vi "RampPointsToArray.vi"(6 "Points":dbl, 9 "Distance":dbl, 10 "Range Z":dbl, 11 "Offset":dbl) -> (2 "RampDistancePoints":dbl[][](array[numeric]), 3 "PointsArray":dbl[](array[numeric]))   [LabVIEW 2016]
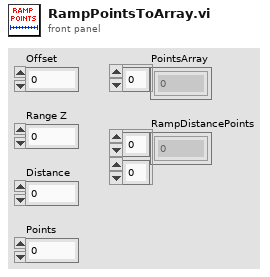
[diagram p1: front panel]
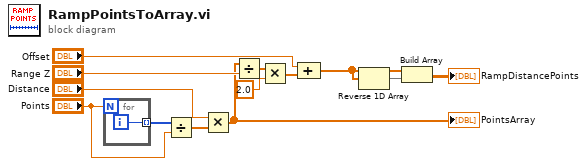
[diagram p0: block diagram]
diagram:
  n1 = for {
    N: "Points" -> [_]
    tunnel: [w14] -> w12 mode=indexing
    i -> [w14]
  }
  n2 = Divide(x=w12, y="Points") -> (x/y=w2:dbl[])
  n3 = Multiply(x="Distance", y=w2) -> (x*y=w10:dbl[])
  "PointsArray" <- w10
  n4 = Divide(x=w10, y="Range Z") -> (x/y=w6:dbl[])
  n5 = Multiply(x=w6, y=2.0) -> (x*y=w9:dbl[])
  n6 = Compound Arithmetic op=ADD("Offset", w9) -> (w5:dbl[])
  n7 = Reverse 1D Array(array=w5) -> (reversed array=w3:dbl[])
  n8 = Build Array(w5, w3) -> (→"RampDistancePoints":dbl[][])
